vi "mix_test.vi"() -> ()   [LabVIEW 2013]
panel:
  in  "signal":i16[](array[numeric])=array[50000 elements]
  in  "Sine out":fxp<+/-,16,0>[][](array[numeric])=array50000x4[200000 elements]
  in  "Cosine out":fxp<+/-,16,0>[][](array[numeric])=array50000x4[200000 elements]
  out "Array 4":fxp<+/-,20,16>[](array[numeric])
  out "Array 2":fxp<+/-,25,19>[](array[numeric])
  out "Array 3":fxp<+/-,20,16>[](array[numeric])
  out "Waveform Graph 2":dbl[](graph)
  out "Waveform Graph":i16[][](graph)
  out "N":i32
  out "Array":u64[](array[numeric])
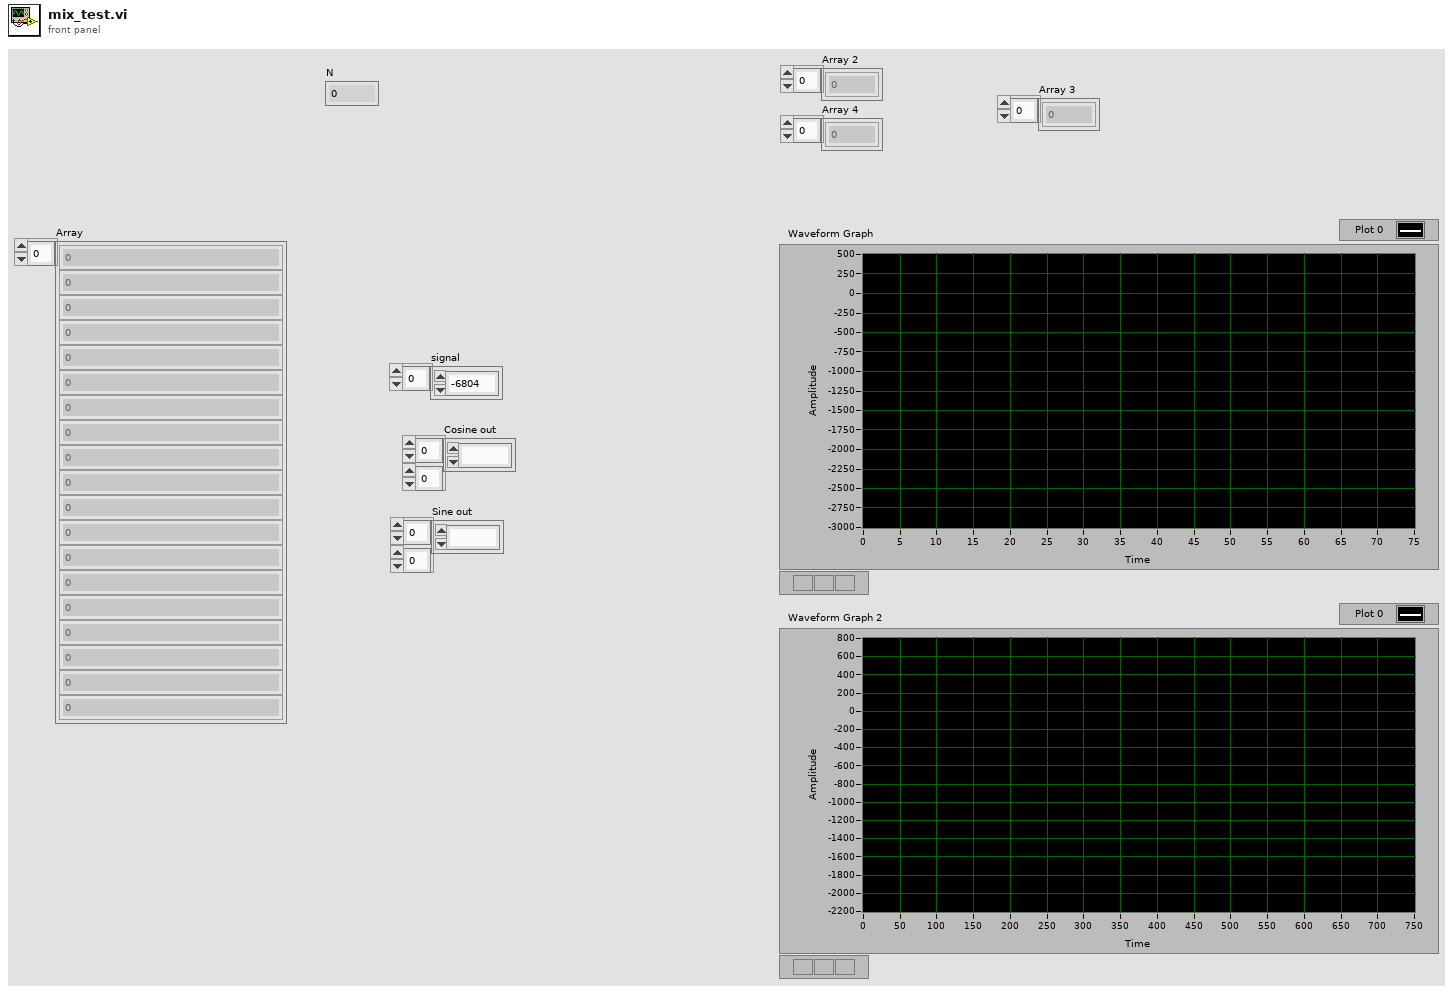
[diagram p1: front panel]
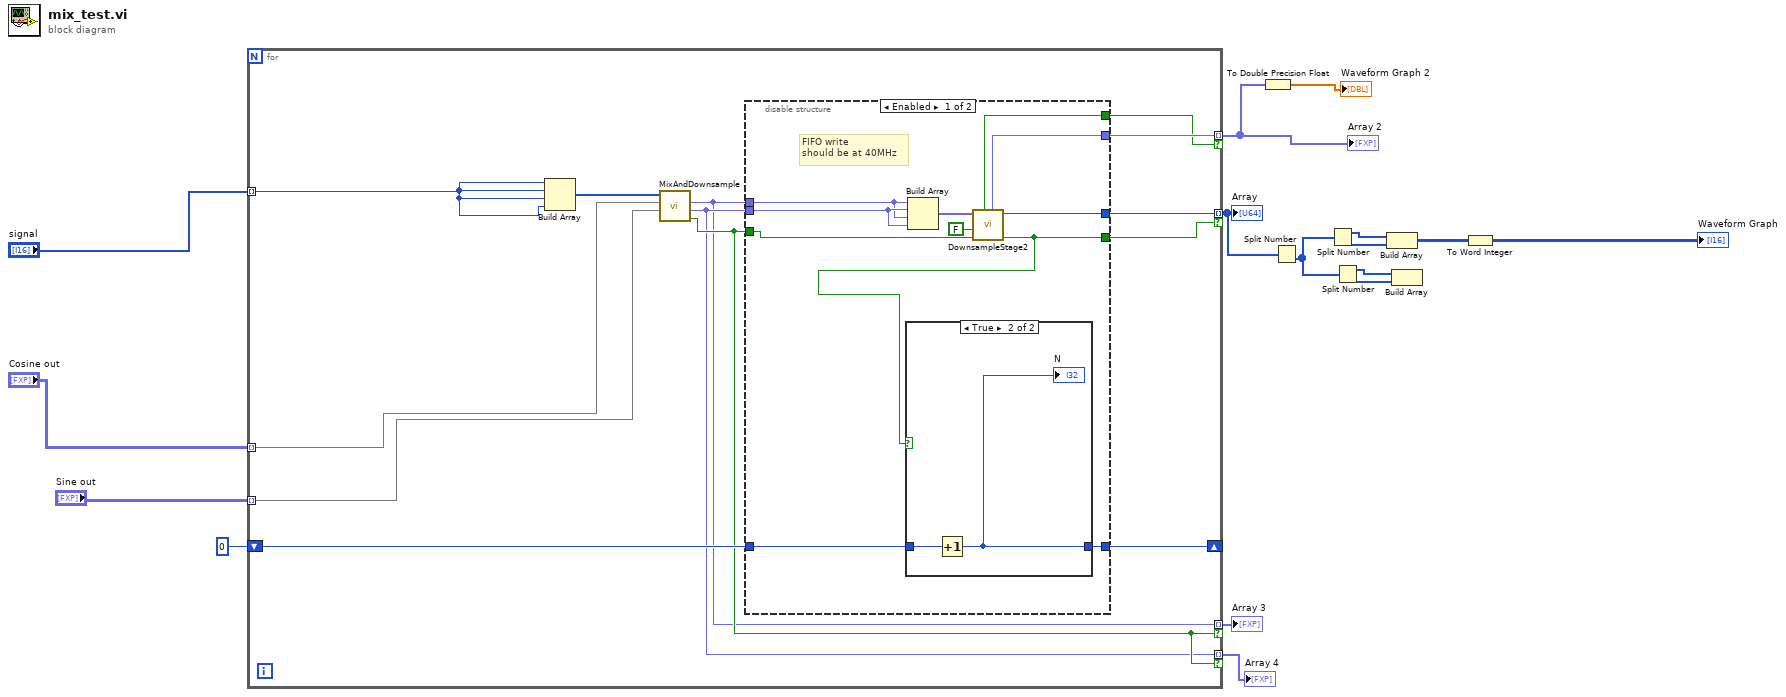
[diagram p0: block diagram]
diagram:
  n1 = for {
    tunnel: [w29] -> w10 mode=indexing if=w17
    shift-right: [w28] -> _
    shift-left: 0 -> [w27]
    tunnel: "Cosine out" -> [w23] mode=indexing
    tunnel: "Sine out" -> [w22] mode=indexing
    tunnel: "signal" -> [w26] mode=indexing
    tunnel: [w19] -> w9 mode=indexing if=w21
    tunnel: [w25] -> w4 mode=indexing if=w18
    tunnel: [w20] -> w8 mode=indexing if=w21
    n2 = Build Array(w26, w26, w26, w26) -> (w24:i16[])
    n3 = call "MixAndDownsample.vi"("Sine in"=w22, "Cosine in"=w23, "Signal Input"=w24) -> ("data valid"=w21:bool, "Q out"=w20:fxp<+/-,20,16>, "I out"=w19:fxp<+/-,20,16>)  [unwired: 6 in]
    n4 = disable-structure shown="Enabled" {
      disable-tunnel: w20 -> [w40 _]
      disable-tunnel: [w39 _] -> w29
      disable-tunnel: [w32 _] -> w17
      disable-tunnel: [w38 _] -> w28
      disable-tunnel: w27 -> [w37 _]
      disable-tunnel: w19 -> [w36 _]
      disable-tunnel: w21 -> [w33 _]
      disable-tunnel: [w35 _] -> w25
      disable-tunnel: [w31 _] -> w18
      frame Enabled {
        # "FIFO write\nshould be at 40MHz"
        n5 = Build Array(w36, w40, w36, w40) -> (w34:fxp<+/-,20,16>[])
        n6 = call "DownsampleStage2.vi"("valid in"=w33, "reset"=FALSE, "Element"=w34) -> ("valid out"=w32:bool, "Element"=w39:u64, "dout"=w35:fxp<+/-,25,19>, "cic valid out"=w31:bool)  [unwired: 5 in]
        n7 = case shown="True" w32 {
          tunnel: [w41 w43] -> w38
          tunnel: w37 -> [w41 w42]
          frame False {
          }
          frame True {
            n8 = Increment(x=w42) -> (x+1=w43:i32)
            "N" <- w43
          }
        }
      }
      frame Disabled {
      }
    }
  }
  "Array" <- w10
  "Array 3" <- w9
  "Array 2" <- w4
  "Array 4" <- w8
  n9 = To Double Precision Float(number=w4) -> (double precision float=→"Waveform Graph 2":dbl[])
  n10 = Split Number(x=w10) -> (lo(x)=w11:u32[])  [unwired: 1 out]
  n11 = Split Number(x=w11) -> (hi(x)=w15:u16[], lo(x)=w14:u16[])
  n12 = Split Number(x=w11) -> (hi(x)=w12:u16[], lo(x)=w13:u16[])
  n13 = Build Array(w15, w14) -> (w2:u16[][])
  n14 = Build Array(w12, w13) -> ()  [unwired: 1 out]
  n15 = To Word Integer(number=w2) -> (16bit integer=→"Waveform Graph":i16[][])
